vi "AlliGator Read HDF5 SSX Detector nformation.vi"(8 "error in (no error)":errorcluster, 11 "ref in":T1 format="%.0x") -> (0 "error out":errorcluster, 3 "SwissSPAD Detector Information":string)   [LabVIEW 2021, in "AlliGator HDF5.lvlib"]
doc: "Reads HDF5 FLI dataset SSx detector information."
uses:
  AlliGator HDF5.lvlib
  <vilib>/addons/h5labview2/base/hid_t.ctl
  <vilib>/addons/h5labview2/base/lib_path.vi
  <vilib>/addons/h5labview2/base/H5Equery.vi
  <vilib>/addons/h5labview2/dataset/H5Dread.llb/H5Dread.xnode
  <vilib>/addons/h5labview2/group/H5G.lvlib
panel:
  # "see the AlliGator License on the block diagram (Ctrl+E or Window:Show Block Diagram)"
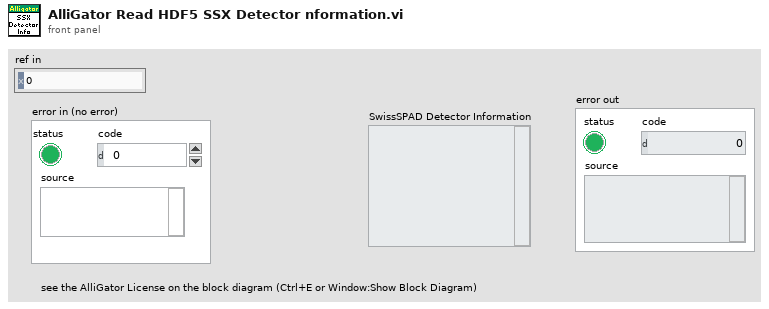
[diagram p1: front panel]
types:
  T1 = typedef "hid_t.ctl" = i64
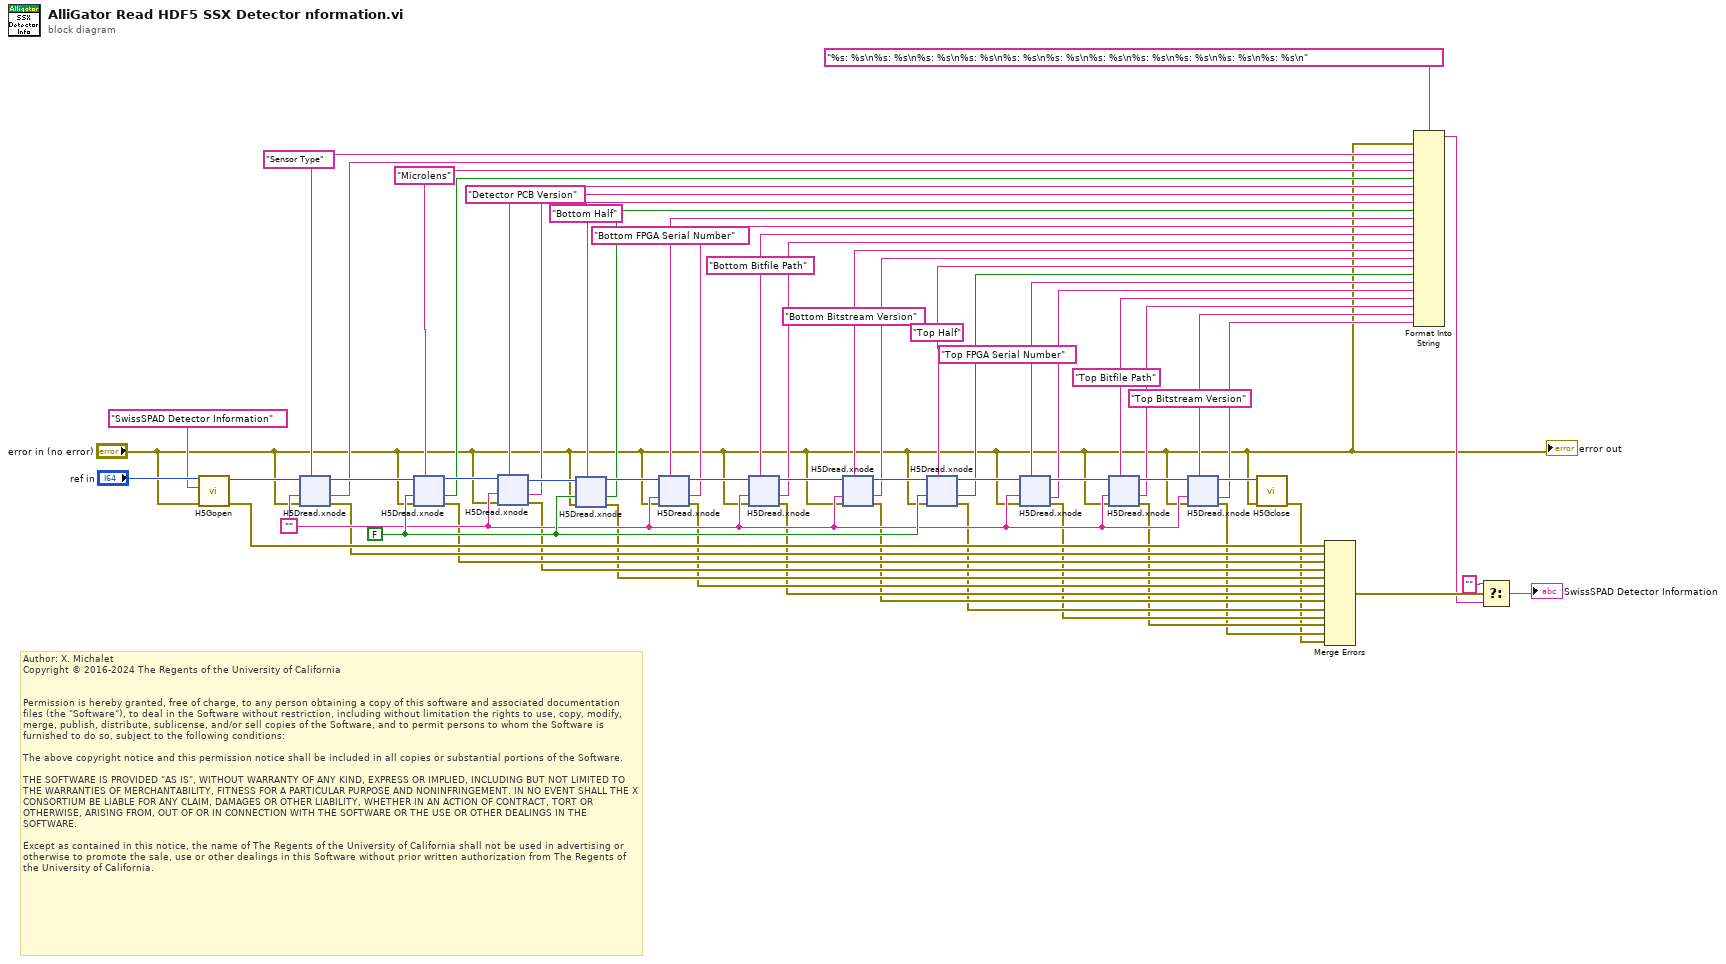
[diagram p0: block diagram]
diagram:
  w43 = ""
  w44 = FALSE
  w13 = "Top Half" ("dataset name")
  w21 = "Bottom Half" ("dataset name")
  w25 = "Microlens" ("dataset name")
  w7 = "Top Bitstream Version" ("dataset name")
  w9 = "Top Bitfile Path" ("dataset name")
  w11 = "Top FPGA Serial Number" ("dataset name")
  w15 = "Bottom Bitstream Version" ("dataset name")
  w17 = "Bottom Bitfile Path" ("dataset name")
  w19 = "Bottom FPGA Serial Number" ("dataset name")
  w23 = "Detector PCB Version" ("dataset name")
  w27 = "Sensor Type" ("dataset name")
  # "Author: X. Michalet\nCopyright © 2016-2024 The Regents of the University of California\n \n\nPermission is hereby granted, free of charge, to any person obtaining a copy of this software and associated documentation files (the \"Software\"), to deal in the Software without restriction, including without limitation the rights to use, copy, modify, merge, publish, distribute, sublicense, and/or sell copies of the Software, and to permit persons to whom the Software is furnished to do so, subject to the following conditions:\n\nThe above copyright notice and this permission notice shall be included in all copies or substantial portions of the Software.\n\nTHE SOFTWARE IS PROVIDED \"AS IS\", WITHOUT WARRANTY OF ANY KIND, EXPRESS OR IMPLIED, INCLUDING BUT NOT LIMITED TO THE WARRANTIES OF MERCHANTABILITY, FITNESS FOR A PARTICULAR PURPOSE AND NONINFRINGEMENT. IN NO EVENT SHALL THE X CONSORTIUM BE LIABLE FOR ANY CLAIM, DAMAGES OR OTHER LIABILITY, WHETHER IN AN ACTION OF CONTRACT, TORT OR OTHERWISE, ARISING FROM, OUT OF OR IN CONNECTION WITH THE SOFTWARE OR THE USE OR OTHER DEALINGS IN THE SOFTWARE.\n\nExcept as contained in this notice, the name of The Regents of the University of California shall not be used in advertising or otherwise to promote the sale, use or other dealings in this Software without prior written authorization from The Regents of the University of California."
  n1 = call <vilib>:"H5Gopen.vi"("error in (no error)"="error in (no error)", "name"="SwissSPAD Detector Information", "ref in"="ref in") -> ("error out"=w42:errorcluster, "group out"=w57:T1)  [unwired: 7 in]
  n2 = xnode "H5Dread.xnode"("dataset name (this)"=w27, "error in (no error)"="error in (no error)", "default"=w43, "ref in"=w57) -> ("error out"=w41:errorcluster, "data"=w26:string, "ref out"=w51:i64)  [unwired: 2 in, 1 out]
  n3 = xnode "H5Dread.xnode"("dataset name (this)"=w25, "error in (no error)"="error in (no error)", "default"=w44, "ref in"=w51) -> ("error out"=w40:errorcluster, "data"=w24:bool, "ref out"=w48:T1)  [unwired: 2 in, 1 out]
  n4 = xnode "H5Dread.xnode"("dataset name (this)"=w23, "error in (no error)"="error in (no error)", "default"=w43, "ref in"=w48) -> ("error out"=w39:errorcluster, "data"=w22:string, "ref out"=w47:T1)  [unwired: 2 in, 1 out]
  n5 = xnode "H5Dread.xnode"("dataset name (this)"=w21, "error in (no error)"="error in (no error)", "default"=w44, "ref in"=w47) -> ("error out"=w38:errorcluster, "data"=w20:bool, "ref out"=w46:T1)  [unwired: 2 in, 1 out]
  n6 = xnode "H5Dread.xnode"("dataset name (this)"=w19, "error in (no error)"="error in (no error)", "default"=w43, "ref in"=w46) -> ("error out"=w37:errorcluster, "data"=w18:string, "ref out"=w56:T1)  [unwired: 2 in, 1 out]
  n7 = xnode "H5Dread.xnode"("dataset name (this)"=w17, "error in (no error)"="error in (no error)", "default"=w43, "ref in"=w56) -> ("error out"=w36:errorcluster, "data"=w16:string, "ref out"=w55:T1)  [unwired: 2 in, 1 out]
  n8 = xnode "H5Dread.xnode"("dataset name (this)"=w15, "error in (no error)"="error in (no error)", "default"=w43, "ref in"=w55) -> ("error out"=w35:errorcluster, "data"=w14:string, "ref out"=w50:T1)  [unwired: 2 in, 1 out]
  n9 = xnode "H5Dread.xnode"("dataset name (this)"=w13, "error in (no error)"="error in (no error)", "default"=w44, "ref in"=w50) -> ("error out"=w34:errorcluster, "data"=w12:bool, "ref out"=w49:T1)  [unwired: 2 in, 1 out]
  n10 = xnode "H5Dread.xnode"("dataset name (this)"=w11, "error in (no error)"="error in (no error)", "default"=w43, "ref in"=w49) -> ("error out"=w33:errorcluster, "data"=w10:string, "ref out"=w54:T1)  [unwired: 2 in, 1 out]
  n11 = xnode "H5Dread.xnode"("dataset name (this)"=w9, "error in (no error)"="error in (no error)", "default"=w43, "ref in"=w54) -> ("error out"=w32:errorcluster, "data"=w8:string, "ref out"=w53:T1)  [unwired: 2 in, 1 out]
  n12 = xnode "H5Dread.xnode"("dataset name (this)"=w7, "error in (no error)"="error in (no error)", "default"=w43, "ref in"=w53) -> ("error out"=w31:errorcluster, "data"=w6:string, "ref out"=w52:T1)  [unwired: 2 in, 1 out]
  n13 = call <vilib>:"H5Gclose.vi"("error in (no error)"="error in (no error)", "group in"=w52) -> ("error out"=w30:errorcluster)  [unwired: 9 in]
  n14 = Merge Errors(w42, w41, w40, w39, w38, w37, w36, w35, w34, w33, w32, w31, w30) -> (w5:errorcluster)
  n15 = Format Into String(format string="%s: %s\n%s: %s\n%s: %s\n%s: %s\n%s: %s\n%s: %s\n%s: %s\n%s: %s\n%s: %s\n%s: %s\n%s: %s\n", error in="error in (no error)", w27, w26, w25, w24, w23, w22, w21, w20, w19, w18, w17, w16, w15, w14, w13, w12, w11, w10, w9, w8, w7, w6) -> (resulting string=w4:string)  [unwired: 1 in, 1 out]
  n16 = Select(t="", s=w5, f=w4) -> (s? t:f=→"SwissSPAD Detector Information":string)
  "error out" <- "error in (no error)"
